vi "GetOutput.vi"(4 "error in":errorcluster, 5 "connection ID":refnum<k5>) -> (0 "Output":string, 1 "error out":errorcluster, 2 "connection ID out":refnum<k5>, 3 "Answer":bool)   [LabVIEW 2013]
panel:
  out "читаю hex":string
  out "читаю текст":string
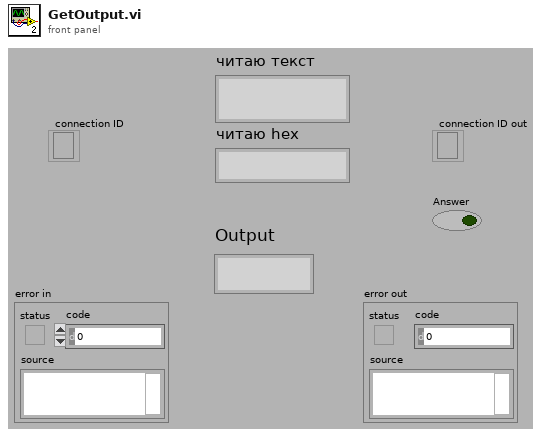
[diagram p1: front panel]
types:
  T1 = enum16{"Standard", "Buffered", "CRLF", "Immediate"}
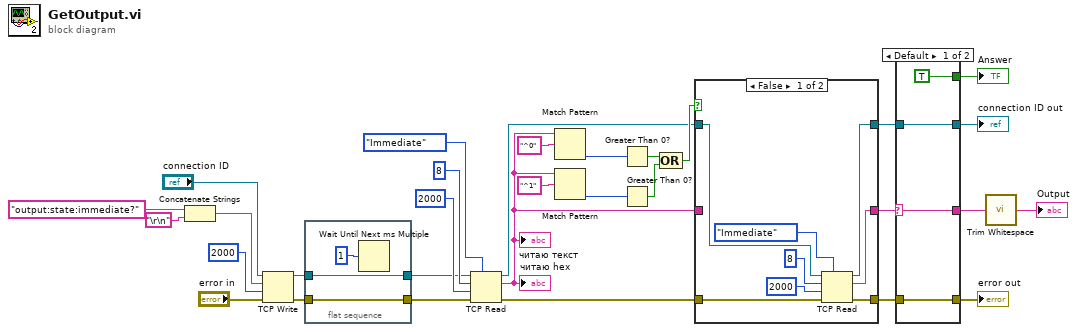
[diagram p0: block diagram]
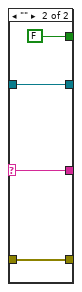
[diagram p3: hidden frame]
diagram:
  n1 = Concatenate Strings("output:state:immediate?" ("data in"), "\r\n") -> (w28:string)
  n2 = TCP Write(connection ID="connection ID", data in=w28, error in (no error)="error in", 9:2000 ("timeout ms (25000)")) -> (connection ID out=w25:refnum<k5>, error out=w26:errorcluster)  [unwired: 1 out]
  n3 = flat-sequence {
    tunnel: [w34] -> w19
    tunnel: w25 -> [w34]
    tunnel: w26 -> [w33]
    tunnel: [w33] -> w20
    frame #0 {
      n4 = Wait Until Next ms Multiple(millisecond multiple=u32 1) -> ()  [unwired: 1 out]
    }
  }
  n5 = TCP Read(connection ID=w19, bytes to read=8, error in (no error)=w20, 7:T1."Immediate" ("mode (standard)"), 9:2000 ("timeout ms (25000)")) -> (connection ID out=w5:refnum<k5>, data out=w2:string, error out=w4:errorcluster)
  "читаю текст" <- w2
  "читаю hex" <- w2
  n6 = Match Pattern(string=w2, regular expression="^0") -> (offset past match=w14:i32)  [unwired: 1 in, 3 out]
  n7 = Match Pattern(string=w2, regular expression="^1") -> (offset past match=w16:i32)  [unwired: 1 in, 3 out]
  n8 = Greater Than 0?(x=w14) -> (x > 0?=w9:bool)
  n9 = Greater Than 0?(x=w16) -> (x > 0?=w8:bool)
  n10 = Compound Arithmetic op=OR(w9, w8) -> (w7:bool)
  n11 = case shown="False" w7 {
    tunnel: [w36 w45] -> w6
    tunnel: w5 -> [w35 w45]
    tunnel: w4 -> [w39 w44]
    tunnel: [w38 w44] -> w3
    tunnel: w2 -> [_ w43]
    tunnel: [w37 w43] -> w1
    frame False {
      n12 = TCP Read(connection ID=w35, bytes to read=8, error in (no error)=w39, 7:T1."Immediate" ("mode (standard)"), 9:2000 ("timeout ms (25000)")) -> (connection ID out=w36:refnum<k5>, data out=w37:string, error out=w38:errorcluster)
    }
    frame True {
    }
  }
  n13 = case shown="Default" w1 {
    selector: w1 -> [w49 w53]
    tunnel: [w49 w53] -> w18
    tunnel: [TRUE FALSE] -> w10
    tunnel: w3 -> [w47 w51]
    tunnel: [w47 w51] -> w12
    tunnel: w6 -> [w46 w50]
    tunnel: [w46 w50] -> w11
    frame Default {
    }
    frame "" {
    }
  }
  "Answer" <- w10
  "connection ID out" <- w11
  "error out" <- w12
  n14 = call <vilib>:"Trim Whitespace.vi"("string"=w18) -> ("trimmed string"=→"Output":string)  [unwired: 1 in]
